vi "EncodersGyroToXY.vi"(8 "Locations to keep":u32=1 min=1, 9 "Angle (degrees)":dbl, 10 "Right Distance":dbl, 11 "Left Distance":dbl) -> (2 "XY Graph":cluster{"X":dbl, "Y":dbl}[](graph), 3 "Location":cluster{dbl, dbl})   [LabVIEW 2016]
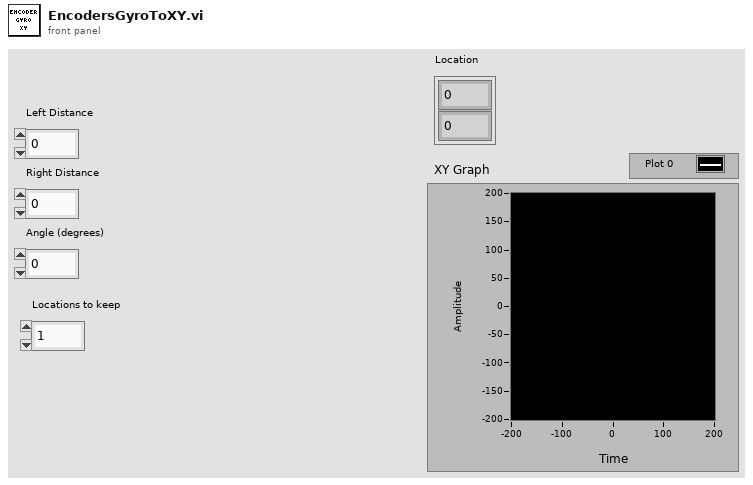
[diagram p1: front panel]
types:
  T1 = cluster{"Sensitivity":dbl, "Sensitivity 2":dbl}[]
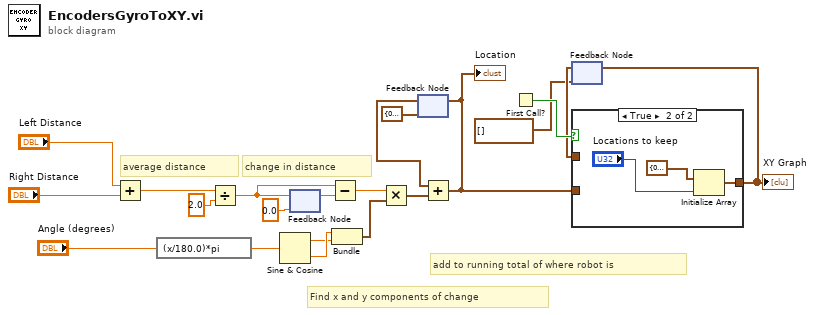
[diagram p0: block diagram]
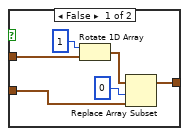
[diagram p2: hidden frame]
diagram:
  # "add to running total of where robot is"
  # "Find x and y components of change"
  # "change in distance"
  # "average distance"
  n1 = Add(x="Left Distance", y="Right Distance") -> (x+y=w3:dbl)
  n2 = expression code="(x/180.0)*pi" ("degrees to radians")("Angle (degrees)") -> (w15:dbl)
  n3 = Divide(x=w3, y=2.0) -> (x/y=w2:dbl)
  n4 = Sine & Cosine(0:w15) -> (1:w13:dbl, 2:w14:dbl)
  n5 = feedback #1(0.0) -> (w18:dbl)
  n6 = feedback-in #1(w2) -> ()
  n7 = Subtract(x=w2, y=w18) -> (x-y=w11:dbl)
  n8 = Bundle(w14, w13) -> (w12:cluster{dbl, dbl})  [unwired: 1 in]
  n9 = Multiply(x=w11, y=w12) -> (x*y=w10:cluster{dbl, dbl})
  n10 = feedback #2(cluster{dbl, dbl} {0.0, 0.0}) -> (w9:cluster{dbl, dbl})
  n11 = Add(x=w9, y=w10) -> (x+y=w8:cluster{dbl, dbl})
  "Location" <- w8
  n12 = feedback-in #2(w8) -> ()
  n13 = First Call?() -> (First Call?: T/F=w21:bool)
  n14 = feedback #3(T1 []) -> (w20:T1)
  n15 = case shown="True" w21 {
    tunnel: [w24 w30] -> w6
    tunnel: w20 -> [w27 _]
    tunnel: w8 -> [w22 _]
    frame False {
      n16 = Rotate 1D Array(1:w27, 2:1 ("n")) -> (0:w25:T1)
      n17 = Replace Array Subset(array=w25, new element=w22, index=0) -> (w24:T1)
    }
    frame True {
      n18 = Initialize Array(cluster{"Sensitivity":dbl, "Sensitivity 2":dbl} {"Sensitivity"=0.0, "Sensitivity 2"=0.0}, "Locations to keep") -> (w30:T1)
    }
  }
  "XY Graph" <- w6
  n19 = feedback-in #3(w6) -> ()
